vi "Handle Command.vi"(8 "error in (no error)":errorcluster, 9 "Data":variant, 10 "Command":string, 11 "Instrument.sample-registry":refnum<class "Instrument.sample-registry.lvclass">) -> (0 "error out":errorcluster, 1 "Processed Data":variant, 2 "Command":string, 3 "Instrument.sample-registry out":refnum<class "Instrument.sample-registry.lvclass">)   [LabVIEW 2019, in "Instrument.sample-registry.lvclass"]
uses:
  Instrument.sample-registry.lvclass
  Instrument.sample-registry.lvclass/Instrument.sample-registry.ctl
  b4d0650f-e901-4c3c-98f8-72e66cea613d.vi
  b4d0650f-e901-4c3c-98f8-72e66cea613d.vi/c60fad33-5b15-4d99-a117-b5456a6e8383.vi
  b4d0650f-e901-4c3c-98f8-72e66cea613d.vi/a731b95d-0a36-40c0-a8b9-a100cbb1949f.vi
  <vilib>/JDP Science/JSONtext/JSON text to Variant.vi
  <vilib>/JDP Science/JSONtext/LVClass Serializer/JSONtext LVClass Serializer.lvclass
  <userlib>/LevyLab/Levylab Instruments/Instrument Types/VSource/Instrument.VSource.lvclass
  cdf0db57-f6bd-4812-9ebb-a5ef629d5d12.vi
  299b1af0-3207-4001-95e1-c675603b2e4b.vi
  3d45e13f-88c6-4418-b8dc-0bfdd8cfd68c.vi
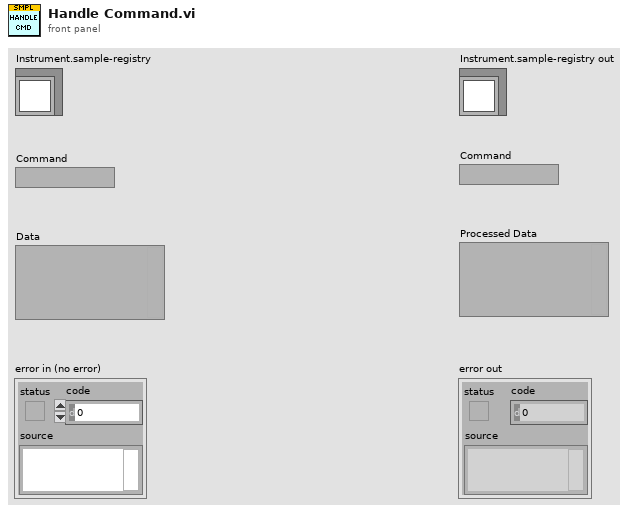
[diagram p1: front panel]
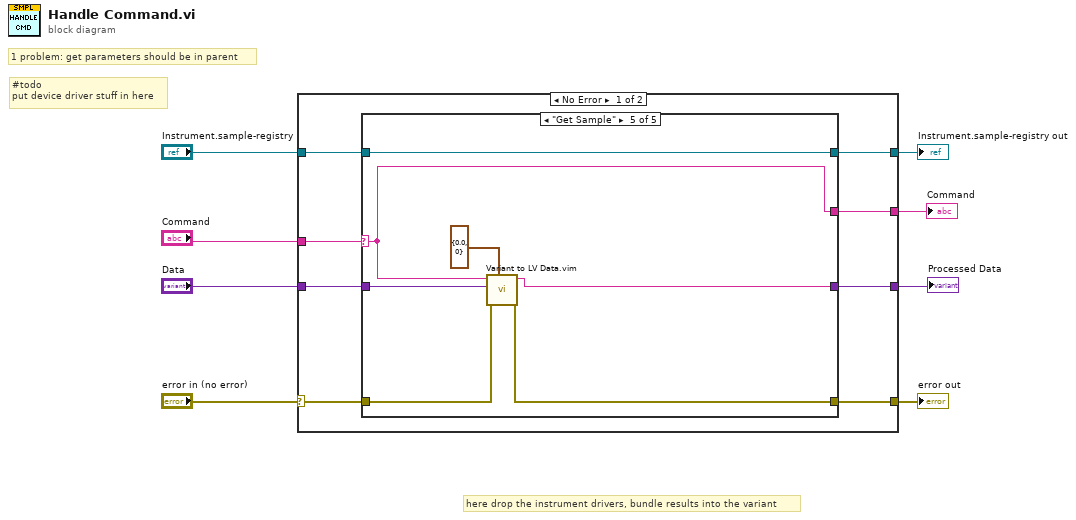
[diagram p0: block diagram]
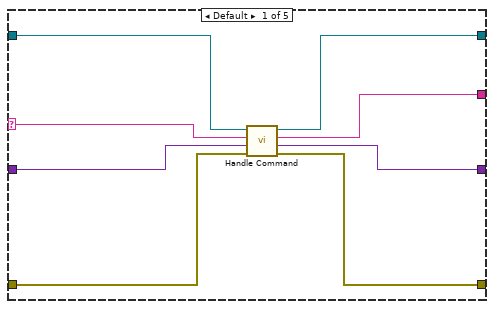
[diagram p2: hidden frame]
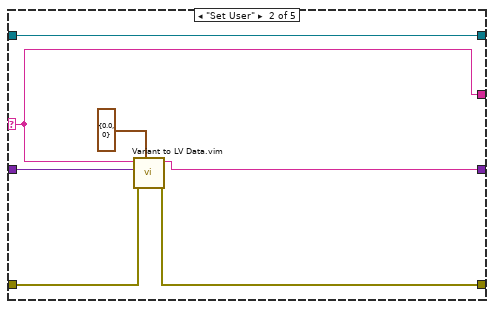
[diagram p3: hidden frame]
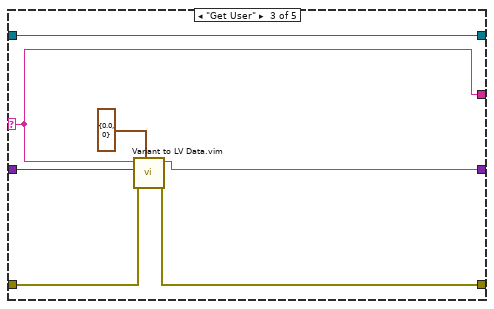
[diagram p4: hidden frame]
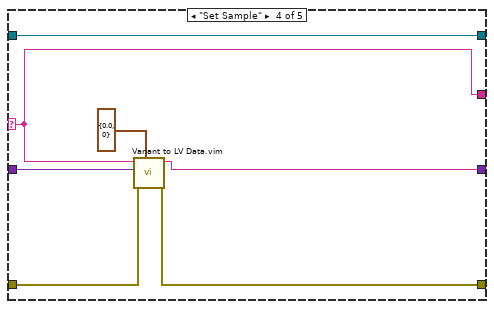
[diagram p5: hidden frame]
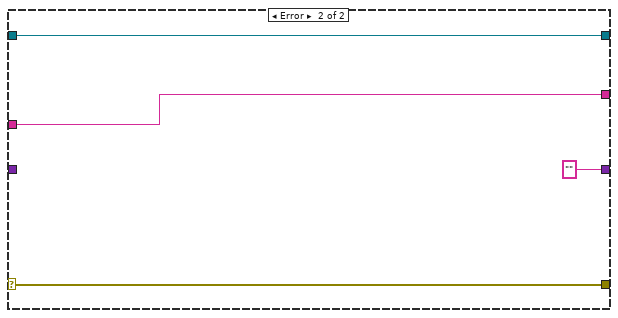
[diagram p6: hidden frame]
diagram:
  # "here drop the instrument drivers, bundle results into the variant"
  # "1 problem: get parameters should be in parent"
  # "#todo\nput device driver stuff in here"
  n1 = case shown="No Error" "error in (no error)" {
    selector: "error in (no error)" -> [w12 w56]
    tunnel: [w10 w56] -> w6
    tunnel: [w14 w55] -> w5
    tunnel: "Instrument.sample-registry" -> [w15 w55]
    tunnel: "Command" -> [w16 w53]
    tunnel: [w13 "" ("String")] -> w3
    tunnel: "Data" -> [w11 _]
    tunnel: [w9 w53] -> w1
    frame No Error {
      n2 = case shown="\"Get Sample\"" w16 {
        selector: w16 -> [w24 w28 w35 w42 w49]
        tunnel: w15 -> [w21 w26 w33 w40 w47]
        tunnel: [w18 w26 w33 w40 w47] -> w14
        tunnel: [w20 w25 w32 w39 w46] -> w13
        tunnel: w12 -> [w22 w30 w37 w44 w51]
        tunnel: w11 -> [w23 w27 w34 w41 w48]
        tunnel: [w19 w29 w36 w43 w50] -> w10
        tunnel: [w17 w28 w35 w42 w49] -> w9
        frame Default {
          n3 = call-parent "Handle Command.vi"("error in (no error)"=w22, "Data"=w23, "Command"=w24, "Instrument in"=w21) -> ("error out"=w19:errorcluster, "Processed Data"=w20:variant, "Command"=w17:string, "Instrument out"=w18:refnum<class "Instrument.sample-registry.lvclass">)  [unwired: 4 in]
        }
        frame "Set User" {
          n4 = call "Variant to LV Data.vim"("type"=cluster{"Bias Voltage (V)":dbl, "Channel":i32} {"Bias Voltage (V)"=0.0, "Channel"=0} ("output cluster"), "error in (no error)"=w30, "Data in"=w27, "Command"=w28) -> ("error out"=w29:errorcluster, "Command out"=w25:string)  [unwired: 4 in, 2 out]
        }
        frame "Get User" {
          n5 = call "Variant to LV Data.vim"("type"=cluster{"Bias Voltage (V)":dbl, "Channel":i32} {"Bias Voltage (V)"=0.0, "Channel"=0} ("output cluster"), "error in (no error)"=w37, "Data in"=w34, "Command"=w35) -> ("error out"=w36:errorcluster, "Command out"=w32:string)  [unwired: 4 in, 2 out]
        }
        frame "Set Sample" {
          n6 = call "Variant to LV Data.vim"("type"=cluster{"Bias Voltage (V)":dbl, "Channel":i32} {"Bias Voltage (V)"=0.0, "Channel"=0} ("output cluster"), "error in (no error)"=w44, "Data in"=w41, "Command"=w42) -> ("error out"=w43:errorcluster, "Command out"=w39:string)  [unwired: 4 in, 2 out]
        }
        frame "Get Sample" {
          n7 = call "Variant to LV Data.vim"("type"=cluster{"Bias Voltage (V)":dbl, "Channel":i32} {"Bias Voltage (V)"=0.0, "Channel"=0} ("output cluster"), "error in (no error)"=w51, "Data in"=w48, "Command"=w49) -> ("error out"=w50:errorcluster, "Command out"=w46:string)  [unwired: 4 in, 2 out]
        }
      }
    }
    frame Error {
    }
  }
  "error out" <- w6
  "Instrument.sample-registry out" <- w5
  "Command" <- w1
  "Processed Data" <- w3
